vi "Adept - Register Write Read.vi"() -> ()   [LabVIEW 2011]
doc: "Write to and read from registers on a Digilent FPGA board."
uses:
  vi.lib/MakerHub/Adept/Private/Type Defs/Adept Device Ctl.xctl
  vi.lib/MakerHub/Adept/Public/Write 1 Register.vi
  vi.lib/MakerHub/Adept/Public/Read 1 Register.vi
  vi.lib/MakerHub/Adept/LVH-Adept.lvlib
panel:
  out "Read Data":u8
  in  "Write Data":u8
  in  "Register Address":u8
  in  "Adept Device":u16(xcontrol)
  # "Configuration"
  # "Write"
  # "Read"
  # "Register Write  / Read\n\nThis example demonstrates how to transfer data to and from\ta Digilent FPGA board.\n\nNote: To use this demonstration, you will need to be connected via USB to a\n\tDigilent FPGA board with the DpimRef design loaded into the gate array.\n\nInstructions\n1. Select the Adept Device.\n2. Enter a Register Address.\n3. Enter a Write Data value\n4. Click the Run Arrow.\n5. The Read Data should match the Write Data."
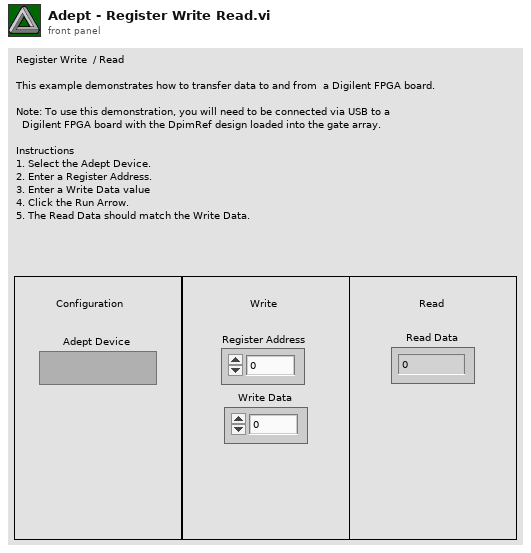
[diagram p1: front panel]
types:
  T1 = typedef "LVH-Adept.lvlib/Device Config.ctl" = cluster{"Num Devices":i32, "Device Names":string[], "Device Index":u16, "Device Handle":u32, "Status":T2}
  T2 = typedef "LVH-Adept.lvlib/Status.ctl" = cluster{"DEPP":bool, "DSTM":bool, "DJTG":bool}
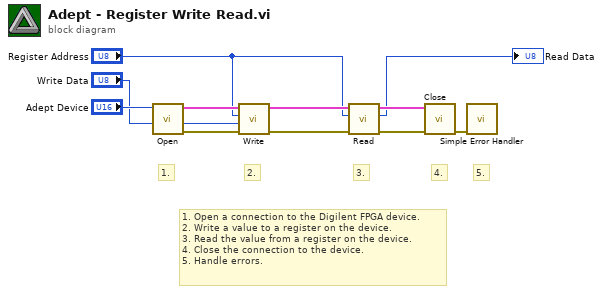
[diagram p0: block diagram]
diagram:
  # "1. Open a connection to the Digilent FPGA device.\n2. Write a value to a register on the device.\n3. Read the value from a register on the device.\n4. Close the connection to the device.\n5. Handle errors."
  # "5."
  # "4."
  # "3."
  # "2."
  # "1."
  n1 = call "Open.vi"("Adept Device"="Adept Device") -> ("Error Out"=w10:errorcluster, "Adept Config"=w11:T1)  [unwired: 9 in]
  n2 = call-poly "Write.vi"("Error In"=w10, "Data"="Write Data", "Register Address"="Register Address", "Adept Config"=w11) -> ("Error Out"=w9:errorcluster, "Adept Config"=w8:T1)  [unwired: 6 in]
  n3 = call-poly "Read.vi"("Error In"=w9, "Register Address"="Register Address", "Adept Config"=w8) -> ("Error Out"=w6:errorcluster, "Data"=→"Read Data":u8, "Adept Config"=w7:T1)  [unwired: 6 in]
  n4 = call "Close.vi"("Error In"=w6, "Adept Config"=w7) -> ("Error Out"=w5:errorcluster)  [unwired: 9 in]
  n5 = call <vilib>:"Simple Error Handler.vi"("error in (no error)"=w5) -> ()  [unwired: 4 in, 5 out]
